vi "CenterOfRotation.vi"(3 "Center of Rotation Joystick Axes":cluster{"X":dbl, "Y":dbl}) -> (0 "Rotation Multipliers":T1, 1 "Rotation Angle Cluster":T2 {"FL Angle" scale=3.1416..-3.1416; "FR Angle" scale=3.1416..-3.1416; "RR Angle" scale=3.1416..-3.1416; "RL Angle" scale=3.1416..-3.1416})   [LabVIEW 2014]
uses:
  Robot Global Data.vi
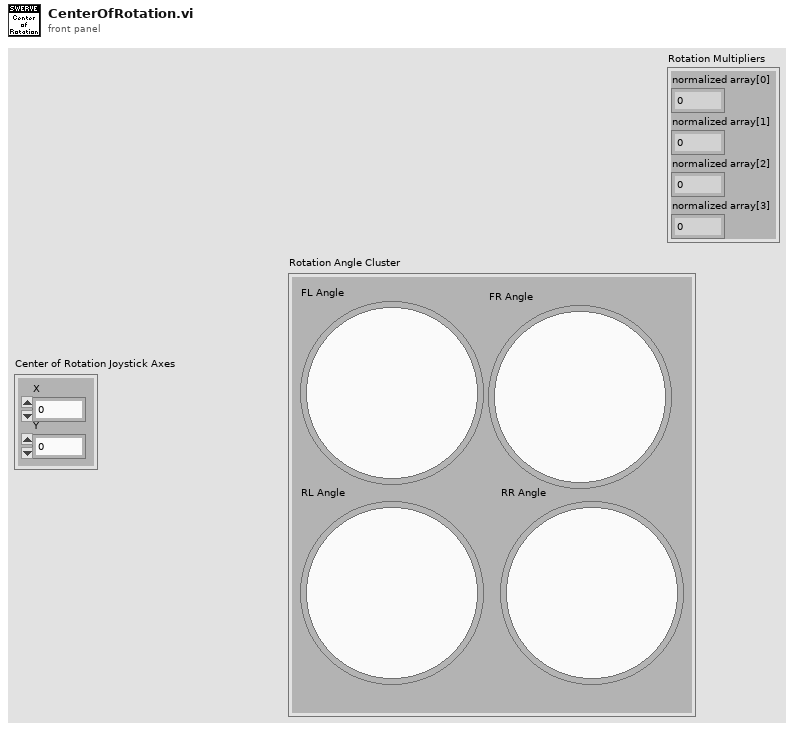
[diagram p1: front panel]
types:
  T1 = cluster{"normalized array[0]":dbl, "normalized array[1]":dbl, "normalized array[2]":dbl, "normalized array[3]":dbl}
  T2 = cluster{"FL Angle":dbl, "FR Angle":dbl, "RL Angle":dbl, "RR Angle":dbl}
  T3 = cluster{"[0]":dbl, "[1]":dbl, "[2]":dbl, "[3]":dbl}
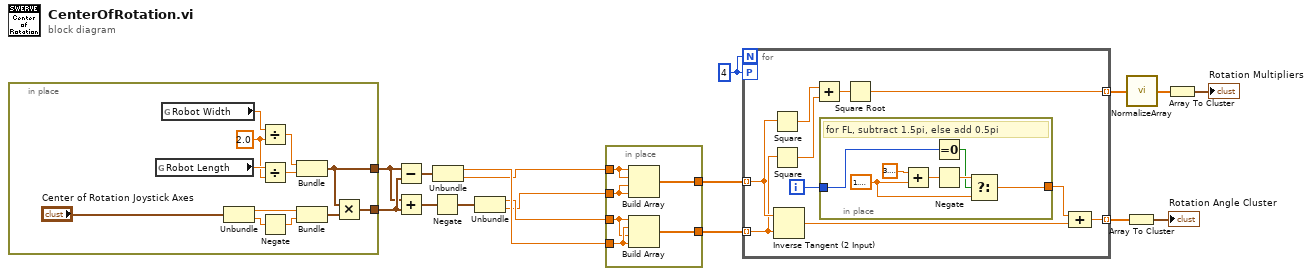
[diagram p0: block diagram]
diagram:
  w7 = 4
  n1 = in-place {
    in-place-border: [w18] -> w14
    in-place-border: [w20] -> w15
    w26 = 2.0 ("y")
    n2 = global read "Robot Global Data.vi" "Robot Length"() -> (w28:dbl)
    n3 = global read "Robot Global Data.vi" "Robot Width"() -> (w27:dbl)
    n4 = Unbundle("Center of Rotation Joystick Axes") -> ("X"=w24:dbl, "Y"=w25:dbl)
    n5 = Divide(x=w27, y=w26) -> (x/y=w22:dbl)
    n6 = Divide(x=w28, y=w26) -> (x/y=w21:dbl)
    n7 = Negate(x=w25) -> (-x=w23:dbl)
    n8 = Bundle(w22, w21) -> (w18:cluster{dbl, dbl})  [unwired: 1 in]
    n9 = Bundle("X"=w24, w23) -> (w19:cluster{"X":dbl, dbl})  [unwired: 1 in]
    n10 = Multiply(x=w18, y=w19) -> (x*y=w20:cluster{dbl, dbl})
  }
  n11 = Subtract(x=w14, y=w15) -> (x-y=w17:cluster{dbl, dbl})
  n12 = Add(x=w14, y=w15) -> (x+y=w16:cluster{dbl, dbl})
  n13 = Negate(x=w16) -> (-x=w4:cluster{dbl, dbl})
  n14 = Unbundle(w17) -> (w13:dbl, w12:dbl)
  n15 = Unbundle(w4) -> (w11:dbl, w10:dbl)
  n16 = in-place {
    in-place-border: w13 -> [w31]
    in-place-border: w12 -> [w35]
    in-place-border: w11 -> [w30]
    in-place-border: w10 -> [w34]
    in-place-border: [w33] -> w9
    in-place-border: [w32] -> w8
    n17 = Build Array(w35, w35, w34, w34) -> (w33:dbl[])
    n18 = Build Array(w30, w31, w30, w31) -> (w32:dbl[])
  }
  n19 = for {
    N: w7 -> [_]
    tunnel: [w41] -> w6 mode=indexing
    tunnel: [w40] -> w3 mode=indexing
    tunnel: w9 -> [w39] mode=indexing
    tunnel: w8 -> [w38] mode=indexing
    workers-P: w7 -> [_]
    i -> [w36]
    n20 = Square(x=w39) -> (x^2=w43:dbl)
    n21 = Square(x=w38) -> (x^2=w42:dbl)
    n22 = Inverse Tangent (2 Input)(1:w38, 2:w39) -> (0:w45:dbl)
    n23 = Add(x=w43, y=w42) -> (x+y=w44:dbl)
    n24 = in-place {
      in-place-border: [w52] -> w37
      in-place-border: w36 -> [w47]
      w51 = 1.5707963267948966
      # "for FL, subtract 1.5pi, else add 0.5pi"
      n25 = Add(x=3.141592653589793, y=w51) -> (x+y=w49:dbl)
      n26 = Equal To 0?(x=w47) -> (x = 0?=w46:bool)
      n27 = Negate(x=w49) -> (-x=w48:dbl)
      n28 = Select(t=w48, s=w46, f=w51) -> (s? t:f=w52:dbl)
    }
    n29 = Square Root(x=w44) -> (sqrt(x)=w40:dbl)
    n30 = Compound Arithmetic op=ADD(w37, w45) -> (w41:dbl)
  }
  n31 = Array To Cluster(array=w6) -> (cluster=→"Rotation Angle Cluster":T3)
  n32 = call "NormalizeArray.vi"("array"=w3) -> ("normalized array"=w2:dbl[])
  n33 = Array To Cluster(array=w2) -> (cluster=→"Rotation Multipliers":T1)
